vi "Status.vi"(8 "error in (no error)":errorcluster, 9 "Return Elements? (T)":bool=TRUE, 11 "Queue in":refnum<queue>) -> (0 "error out":errorcluster, 1 "Data":string[](array[string]), 2 "Messages":string[](array[string]), 3 "Queue out":refnum<queue>, 4 "# Elements in Queue":i32, 5 "Queue Name":string, 6 "Elements":string[](array[string]), 7 "Max Size":i32)   [LabVIEW 2021, in "Queue.lvlib"]
doc: "Returns the status of a queue. If <b>Return Elements?</b> is True, this returns the `<msg>,<data>` element parts."
uses:
  Queue.lvlib
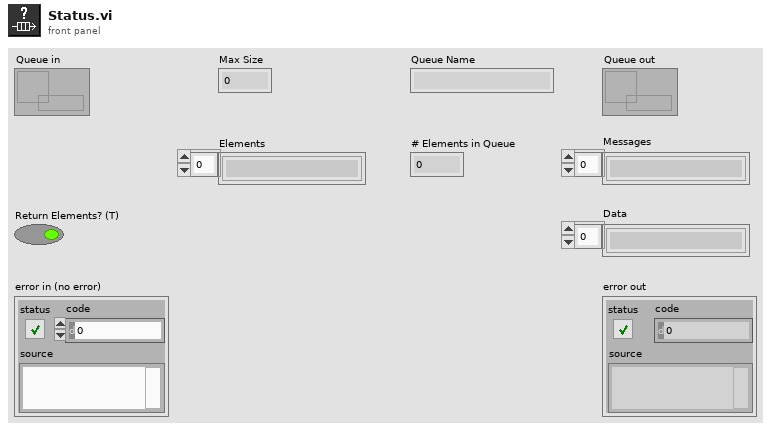
[diagram p1: front panel]
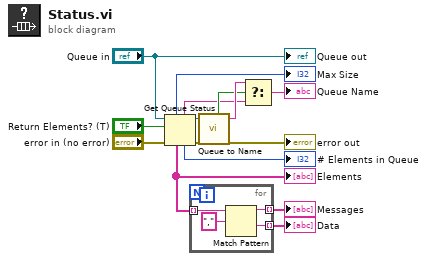
[diagram p0: block diagram]
diagram:
  n1 = Get Queue Status(queue="Queue in", return elements? (F)="Return Elements? (T)", error in (no error)="error in (no error)") -> (queue out=w5:refnum<queue>, queue name=w2:string, max queue size=→"Max Size":i32, error out=→"error out":errorcluster, # elements in queue=→"# Elements in Queue":i32, elements=w8:string[])  [unwired: 2 out]
  "Elements" <- w8
  n2 = for {
    tunnel: [w17] -> w10 mode=indexing
    tunnel: [w15] -> w9 mode=indexing
    tunnel: w8 -> [w16] mode=indexing
    n3 = Match Pattern(string=w16, regular expression=",") -> (before substring=w15:string, after substring=w17:string)  [unwired: 1 in, 2 out]
  }
  "Messages" <- w9
  "Data" <- w10
  n4 = call "Queue to Name.vi"("Queue in"=w5) -> ("Found?"=w3:bool, "Queue Name out"=w4:string)  [unwired: 7 in]
  n5 = Select(t=w4, s=w3, f=w2) -> (s? t:f=→"Queue Name":string)
  "Queue out" <- "Queue in"
